vi "Launch Subordinate Object.vi"(8 "error in (no error)":errorcluster, 9 "Name":string, 10 "Subordinate Object":refnum<class "Template Module.lvclass">, 11 "Measure Object in":refnum<class "Template Module.lvclass">) -> (0 "error out":errorcluster, 2 "Nested Actor's Enqueuer":refnum<class "Message Enqueuer.lvclass">, 3 "Measure Object out":refnum<class "Template Module.lvclass">)   [LabVIEW 2016, in "Template Module.lvclass"]
uses:
  Template Module.lvclass
  <vilib>/ActorFramework/Actor/Actor.lvclass
  C:/Program Files/National Instruments/LabVIEW 2016/vi.lib/ActorFramework/Actor/Actor.lvclass
  <vilib>/ActorFramework/Message Enqueuer/Message Enqueuer.lvclass
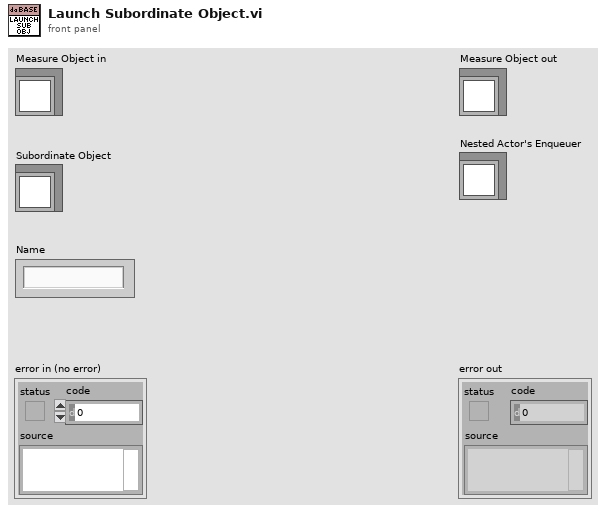
[diagram p1: front panel]
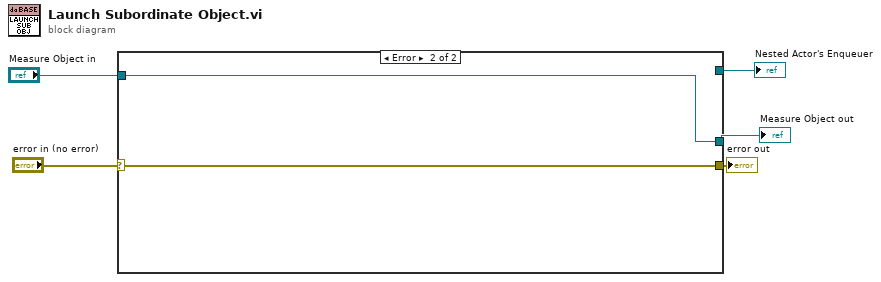
[diagram p0: block diagram]
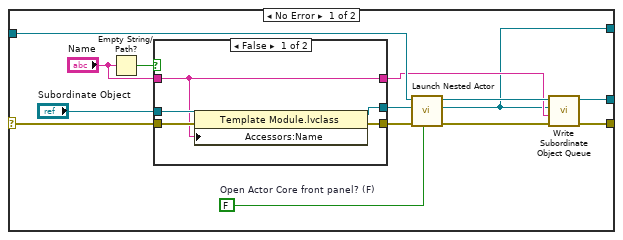
[diagram p2: hidden frame]
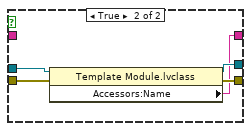
[diagram p3: hidden frame]
diagram:
  n1 = case shown="Error" "error in (no error)" {
    selector: "error in (no error)" -> [w18 w31]
    tunnel: [w10 w31] -> w4
    tunnel: [w13 w30] -> w2
    tunnel: "Measure Object in" -> [w12 w30]
    tunnel: [w6 _] -> w1
    frame No Error {
      w15 = FALSE  # Open Actor Core front panel? (F)
      n2 = Empty String/Path?(string/path="Name") -> (empty?=w8:bool)
      n3 = case shown="False" w8 {
        tunnel: "Subordinate Object" -> [w24 w29]
        tunnel: w18 -> [w23 w28]
        tunnel: [w22 w27] -> w17
        tunnel: [w21 w26] -> w16
        tunnel: "Name" -> [w20 _]
        tunnel: [w20 w25] -> w7
        frame False {
          n4 = property class="Template Module.lvclass"(reference=w24, error in=w23, "Accessors:Name"=w20) -> (reference out=w21:refnum<class "Template Module.lvclass">, error out=w22:errorcluster)
        }
        frame True {
          n5 = property class="Template Module.lvclass"(reference=w29, error in=w28) -> (reference out=w26:refnum<class "Template Module.lvclass">, error out=w27:errorcluster, "Accessors:Name"=w25:string)
        }
      }
      n6 = call <vilib>:"Launch Nested Actor.vi"("Open Actor Core front panel? (F)"=w15, "error in (no error)"=w17, "Nested Actor"=w16, "Caller Actor in"=w12) -> ("error out"=w14:errorcluster, "Nested Actor's Enqueuer"=w6:refnum<class "Message Enqueuer.lvclass">, "Caller Actor out"=w11:refnum<class "Template Module.lvclass">)  [unwired: 5 in]
      n7 = call-dynamic "Write Subordinate Object Queue.vi"("error in (no error)"=w14, "Name"=w7, "Caller-To-Actor Enqueuer"=w6, "Measure Object in"=w11) -> ("error out"=w10:errorcluster, "Measure Object out"=w13:refnum<class "Template Module.lvclass">)  [unwired: 6 in]
    }
    frame Error {
    }
  }
  "error out" <- w4
  "Measure Object out" <- w2
  "Nested Actor's Enqueuer" <- w1
